vi "Write Associated GUI Class.vi"(8 "Error In":errorcluster, 10 "Associated GUI Class":string, 11 "Launch Associated GUI Msg in":refnum<class "Launch Associated GUI Msg.lvclass">) -> (0 "Error Out":errorcluster, 3 "Launch Associated GUI Msg out":refnum<class "Launch Associated GUI Msg.lvclass">)   [LabVIEW 2014, in "CS++BaseActor.lvlib" / "Launch Associated GUI Msg.lvclass"]
doc: "Write DefaultGUI to attribute."
uses:
  Launch Associated GUI Msg.lvclass
  Launch Associated GUI Msg.lvclass/Launch Associated GUI Msg.ctl
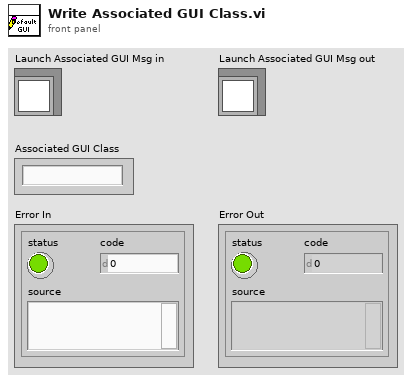
[diagram p1: front panel]
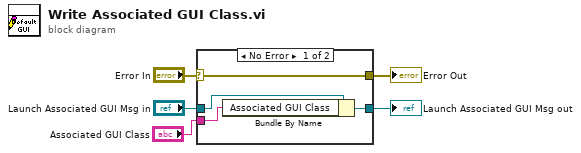
[diagram p0: block diagram]
diagram:
  n1 = case shown="No Error" "Error In" {
    selector: "Error In" -> [w9 w10]
    tunnel: [w9 w10] -> w4
    tunnel: [w7 w11] -> w2
    tunnel: "Launch Associated GUI Msg in" -> [w8 w11]
    tunnel: "Associated GUI Class" -> [w6 _]
    frame No Error {
      n2 = Bundle By Name(cluster=w8, "Associated GUI Class"=w6) -> (w7:refnum<class "Launch Associated GUI Msg.lvclass">)
    }
    frame Error {
    }
  }
  "Error Out" <- w4
  "Launch Associated GUI Msg out" <- w2
